vi "DPT Build DBL Arrry FIFO.vi"(7 "Max Size":i32, 9 "Initialize":bool, 10 "Numeric":dbl) -> (2 "FIFO Array":dbl[](array[numeric]))   [LabVIEW 2016]
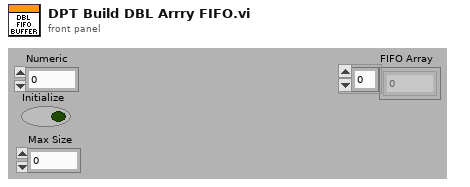
[diagram p1: front panel]
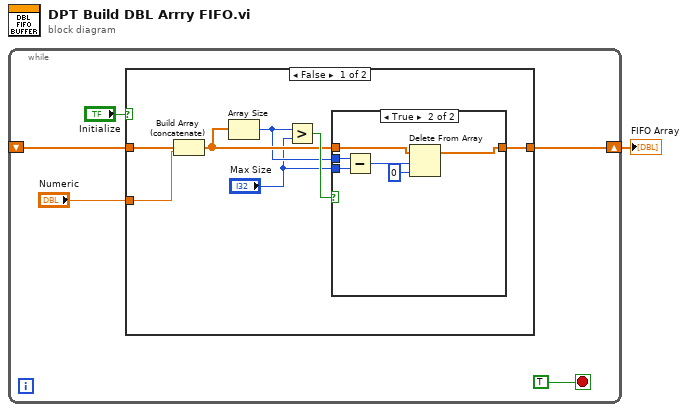
[diagram p0: block diagram]
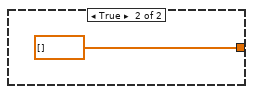
[diagram p3: hidden frame]
diagram:
  n1 = while {
    shift-right: [w4] -> w1
    shift-left: _ -> [w3]
    stop <- TRUE stop-if-true
    n2 = case shown="False" "Initialize" {
      tunnel: "Numeric" -> [w13 _]
      tunnel: [w10 dbl[] []] -> w4
      tunnel: w3 -> [w12 _]
      frame False {
        n3 = Build Array (concatenate)(w12, w13) -> (w9:dbl[])
        n4 = Array Size(array=w9) -> (size(s)=w8:i32)
        n5 = Greater?(x=w8, y="Max Size") -> (0:w11:bool)
        n6 = case shown="True" w11 {
          tunnel: [w14 w19] -> w10
          tunnel: w9 -> [w14 w20]
          tunnel: w8 -> [_ w16]
          tunnel: "Max Size" -> [_ w15]
          frame False {
          }
          frame True {
            n7 = Subtract(x=w16, y=w15) -> (x-y=w17:i32)
            n8 = Delete From Array(array=w20, length=w17, index=0) -> (array with subset deleted=w19:dbl[])  [unwired: 1 out]
          }
        }
      }
      frame True {
      }
    }
  }
  "FIFO Array" <- w1
